vi "PROPERTY NODE.vi"() -> ()   [LabVIEW 2018]
panel:
  in  "Front Panel Window:Closeable":bool
  out "Visible":bool
  out "Numeric 2":i32
  in  "Numeric":i32
  in  "Blinking":bool
  in  "stop":bool
  out "Boolean":bool
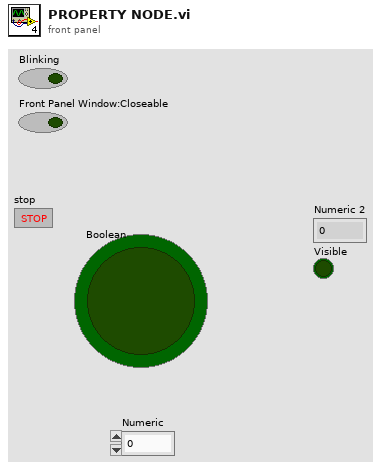
[diagram p1: front panel]
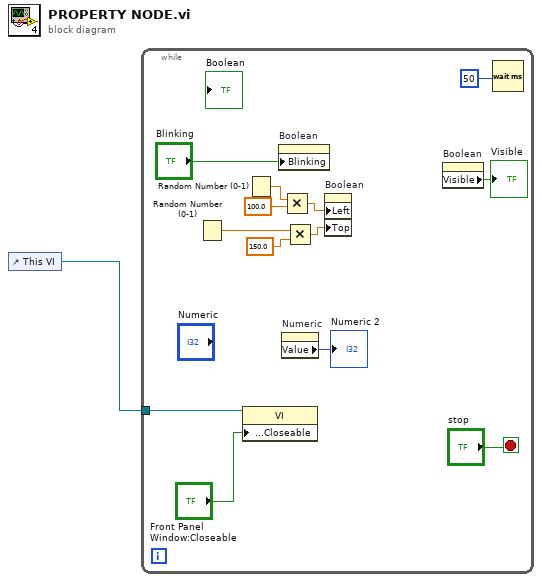
[diagram p0: block diagram]
diagram:
  n1 = control-ref of="This VI"() -> (w1:refnum<vi>)
  n2 = while {
    tunnel: w1 -> [w3]
    stop <- "stop" stop-if-true
    n3 = Random Number (0-1)() -> (number: 0 to 1=w8:dbl)
    n4 = property class="VI"(reference=w3, "Front Panel.Closeable"="Front Panel Window:Closeable") -> ()  [unwired: 1 in, 2 out]
    n5 = Random Number (0-1)() -> (number: 0 to 1=w11:dbl)
    n6 = property on="Boolean" class="Bool (strict)"("Blinking"="Blinking") -> ()  [unwired: 2 in, 2 out]
    n7 = Multiply(x=w11, y=100.0) -> (x*y=w12:dbl)
    n8 = property on="Numeric" class="DigNum (strict)"() -> ("Value"=→"Numeric 2":i32)  [unwired: 2 in, 2 out]
    n9 = Multiply(x=w8, y=150.0) -> (x*y=w9:dbl)
    n10 = property on="Boolean" class="Bool (strict)"("Left"=w12, "Top"=w9) -> ()  [unwired: 2 in, 2 out]
    n11 = property on="Boolean" class="Bool (strict)"() -> ("Visible"=→"Visible":bool)  [unwired: 2 in, 2 out]
    n12 = Wait (ms)(milliseconds to wait=u32 50) -> ()  [unwired: 1 out]
  }
